vi "Read Configuration.vi"(8 "error in (no error)":errorcluster, 11 "Execution UI In":refnum<class "Execution UI V2.lvclass">) -> (0 "error out":errorcluster, 3 "Execution UI Out":refnum<class "Execution UI V2.lvclass">)   [LabVIEW 2020, in "Execution UI V2.lvclass"]
doc: "Method that read any necessay configurations from config file or potentially configure hard coded values. The specified configuration file is validated and loaded."
uses:
  Execution UI V2.lvclass
  Execution UI V2.lvclass/Execution UI V2.ctl
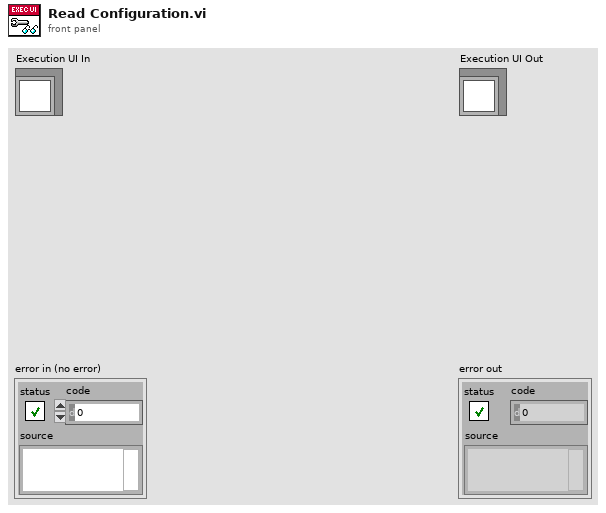
[diagram p1: front panel]
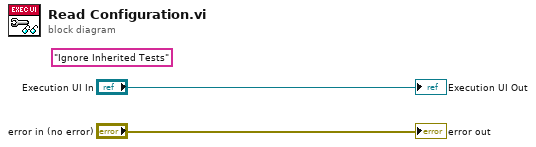
[diagram p0: block diagram]
diagram:
  (unwired) "Ignore Inherited Tests" ("key")
  "error out" <- "error in (no error)"
  "Execution UI Out" <- "Execution UI In"
